vi "GetDataFromLogfile.vi"(11 "appended path":path) -> (2 "Index Values":T1, 3 "Logging":string[][](table))   [LabVIEW 2012]
uses:
  <vilib>/Utility/miscctls.llb/LVRowAndColumnUnsignedTypeDef.ctl
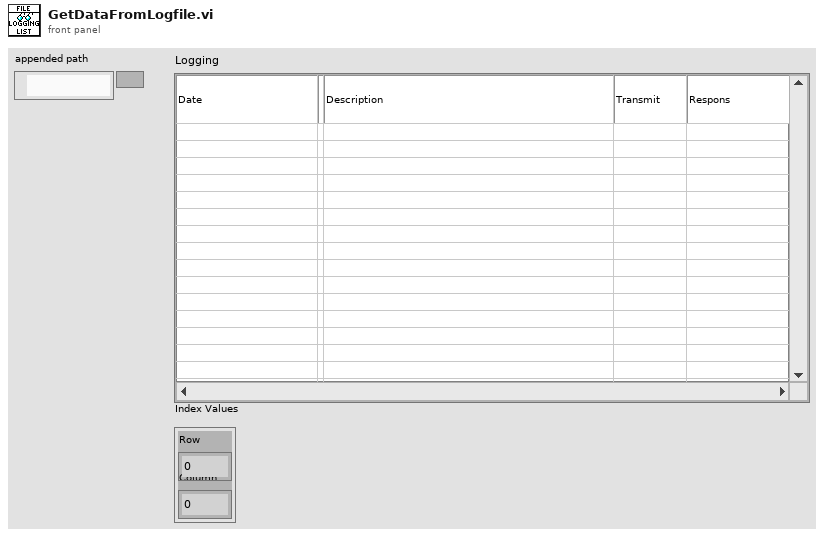
[diagram p1: front panel]
types:
  T1 = typedef "LVRowAndColumnUnsignedTypeDef.ctl" = cluster{"Row":u32, "Column":u32}
  T2 = enum16{"open", "replace", "create", "open or create", "replace or create", "replace or create with confirmation"}
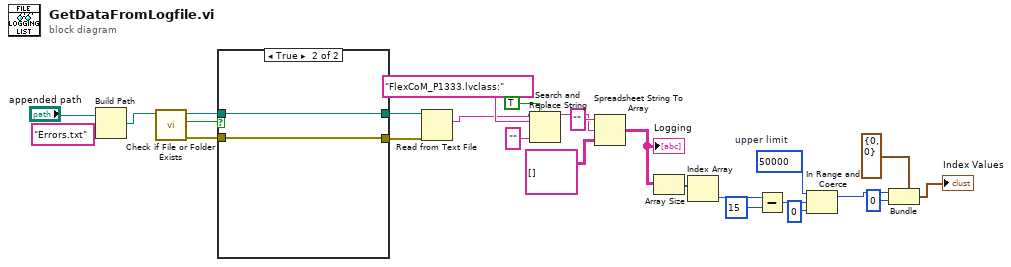
[diagram p0: block diagram]
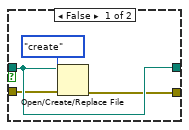
[diagram p2: hidden frame]
diagram:
  w26 = 50000  # upper limit
  n1 = Build Path(base path="appended path", name or relative path="Errors.txt" ("standard input")) -> (appended path=w6:path)
  n2 = call <vilib>:"Check if File or Folder Exists.vi"("path"=w6) -> ("error out"=w2:errorcluster, "file or folder exists?"=w5:bool, "dup path"=w4:path)  [unwired: 8 in]
  n3 = case shown="True" w5 {
    tunnel: w4 -> [w29 w32]
    tunnel: [w29 w32] -> w3
    tunnel: w2 -> [w28 w31]
    tunnel: [w27 w31] -> w1
    frame False {
      n4 = Open/Create/Replace File(file path (use dialog)=w29, error in=w28, operation (0:open)=T2."create") -> (error out=w27:errorcluster)  [unwired: 3 in, 2 out]
    }
    frame True {
    }
  }
  n5 = Read from Text File(file (use dialog)=w3, error in=w1) -> (text=w10:string)  [unwired: 2 in, 3 out]
  n6 = Search and Replace String(replace all?=TRUE ("replace all? (F)"), input string=w10, search string="FlexCoM_P1333.lvclass:", replace string="" ("replace string (\"\")")) -> (result string=w13:string)  [unwired: 4 in, 3 out]
  n7 = Spreadsheet String To Array(format string="", spreadsheet string=w13, array type (2D Dbl)=string[][] [] ("Logging")) -> (array=w7:string[][])  [unwired: 1 in]
  "Logging" <- w7
  n8 = Array Size(array=w7) -> (size(s)=w17:i32[])
  n9 = Index Array(array=w17) -> (element=w22:i32)  [unwired: 1 in]
  n10 = Subtract(x=w22, y=15) -> (x-y=w24:i32)
  n11 = In Range and Coerce(upper limit=w26, x=w24, lower limit=0 ("y")) -> (coerced(x)=w23:i32)  [unwired: 1 out]
  n12 = Bundle(cluster=T1 {"Row"=0, "Column"=0} ("Index Values"), "Row"=w23, "Column"=u32 0) -> (→"Index Values":T1)
